vi "Line Intersection With Sprite.vi"(9 "Pixel Data in":u32[][](array[colorbox]), 10 "Line End Point":refnum<class "Vector 2D.lvclass">, 11 "Line Start Point":refnum<class "Vector 2D.lvclass">) -> (2 "Hit Point":refnum<class "Vector 2D.lvclass">, 3 "Hit":bool)   [LabVIEW 2021, in "Collision.lvlib"]
uses:
  Collision.lvlib
  Vector 2D/Vector 2D.lvclass
  Vector 2D/Vector 2D.lvclass/Vector 2D.ctl
panel:
  out "Pixel Data out":u32[][](array[colorbox])
  in  "Colour":u32(colorbox)=16720402
  out "Iteration":i32
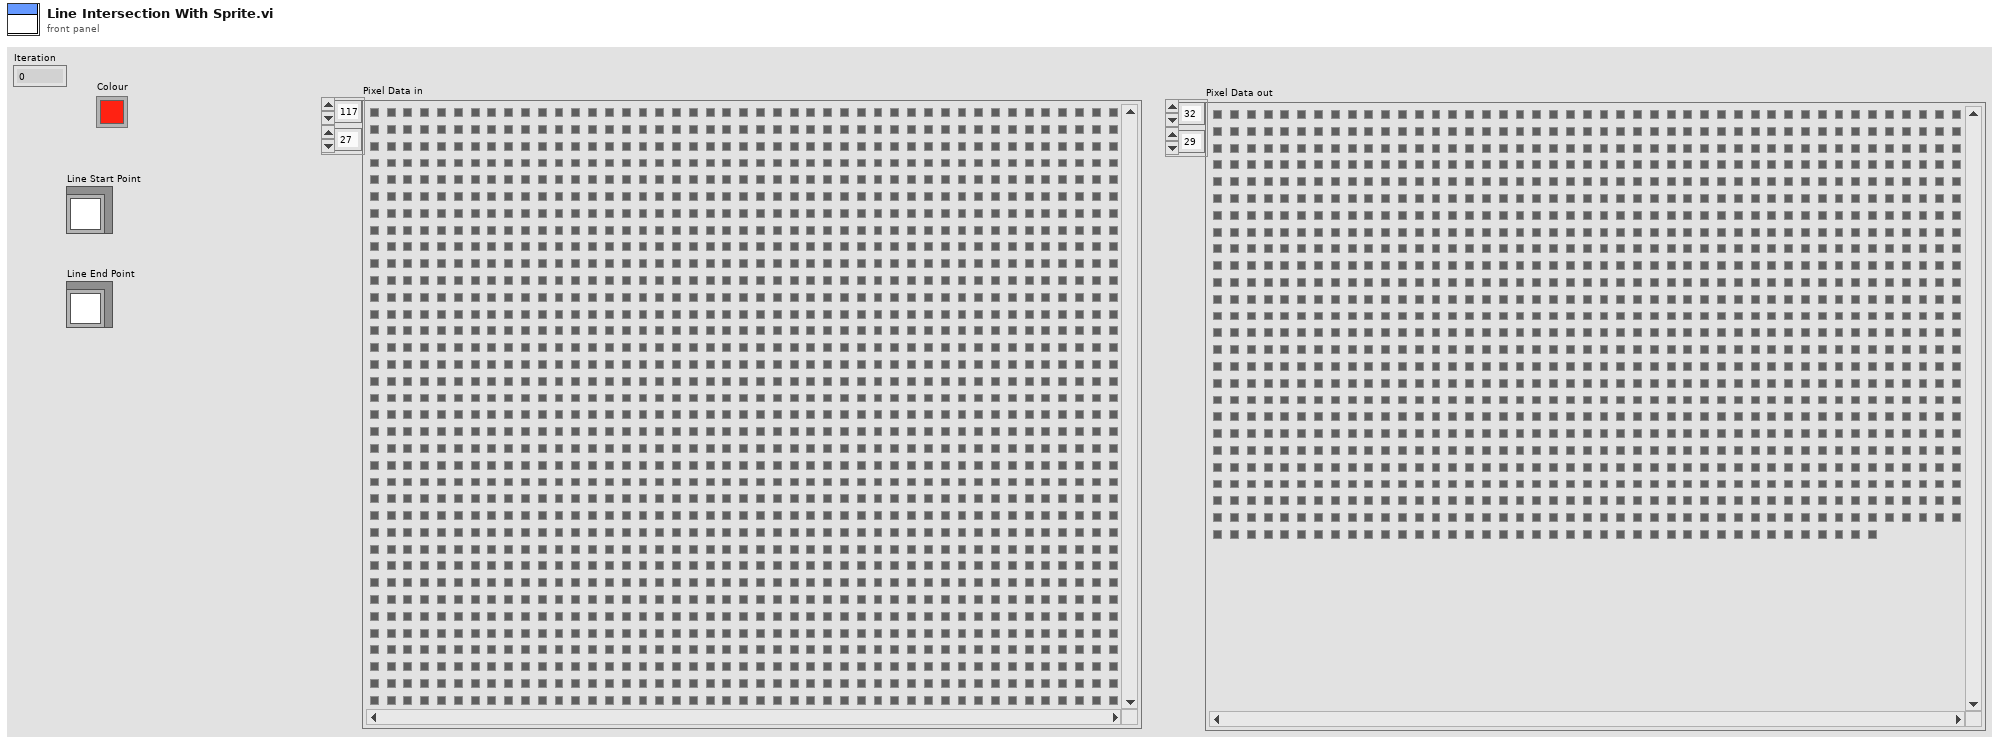
[diagram p1: front panel]
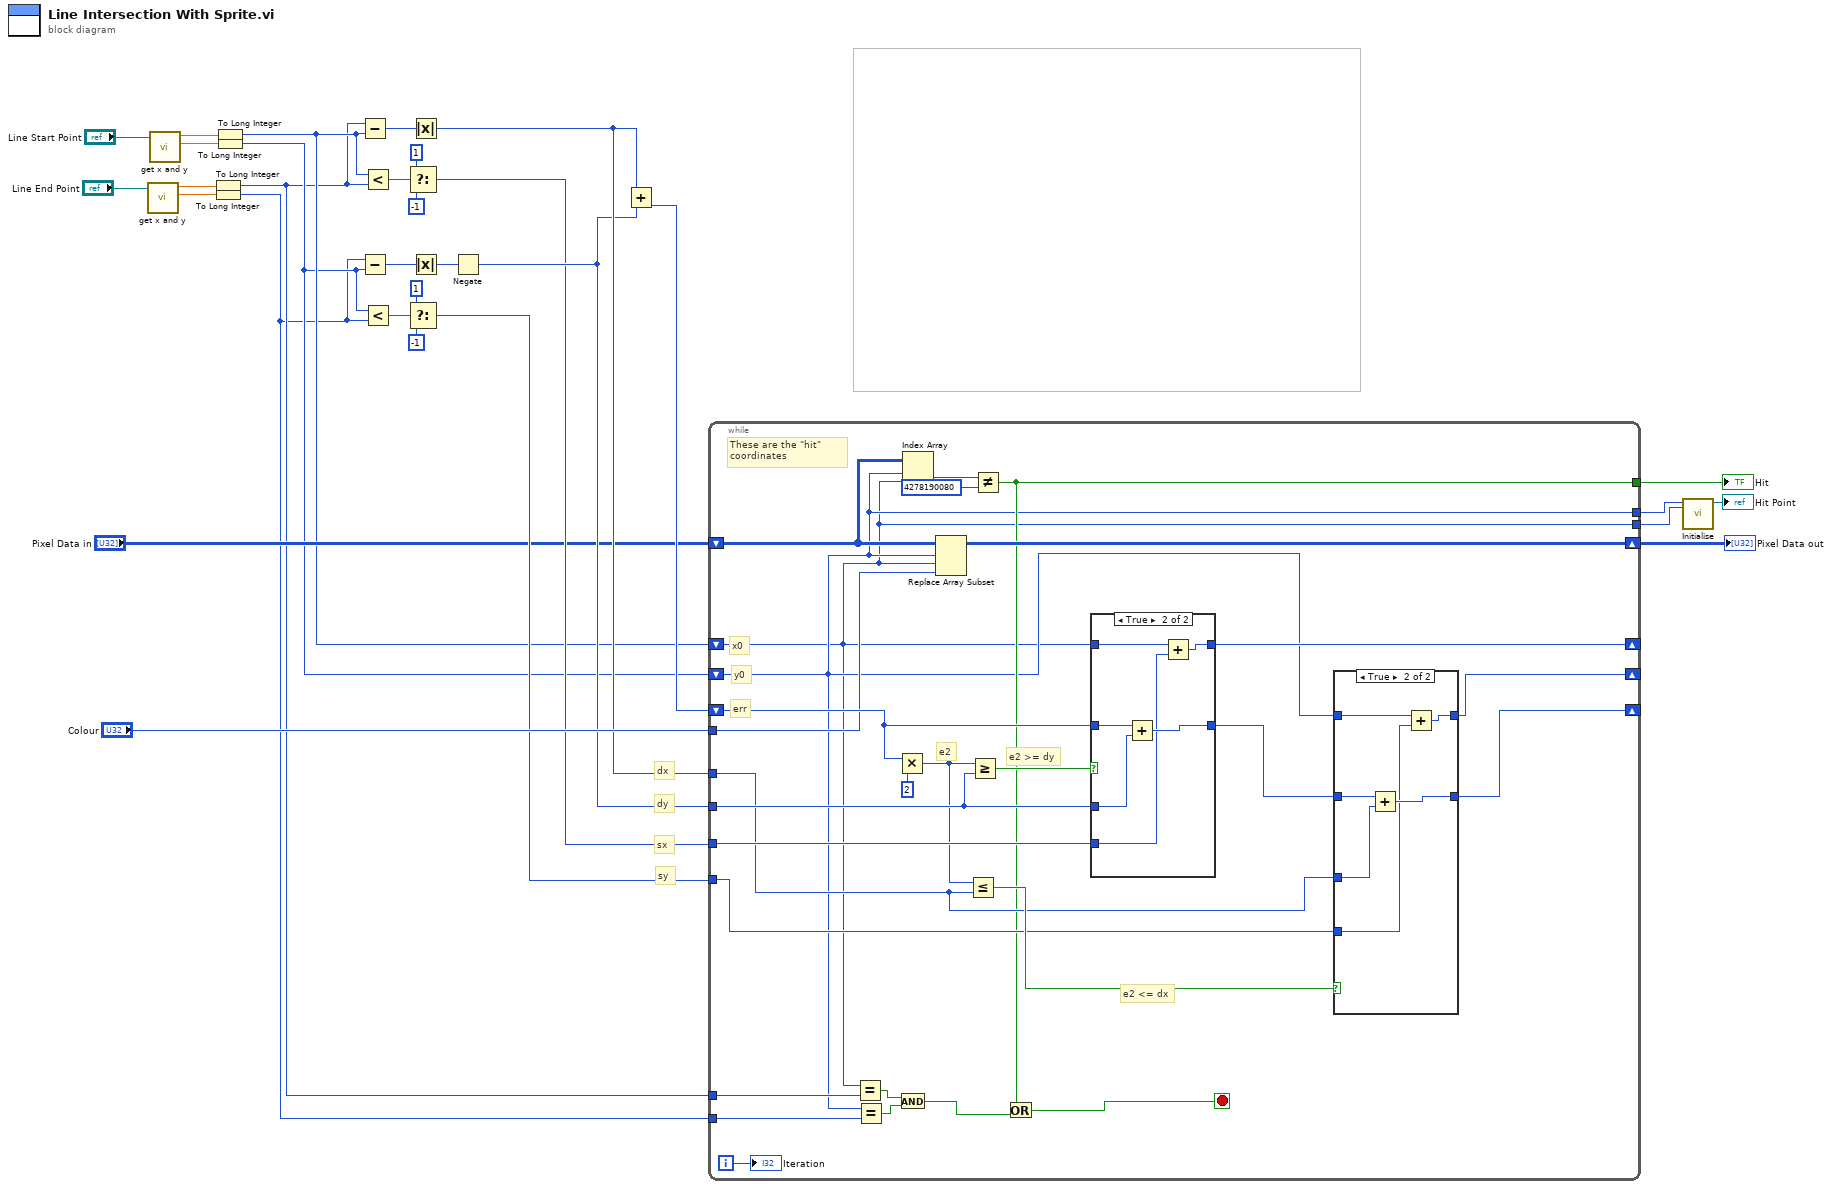
[diagram p0: block diagram]
diagram:
  # "sy"
  # "sx"
  # "dy"
  # "dx"
  n1 = call "get x and y.vi"("Vector 2D in"="Line End Point") -> ("y"=w12:sgl, "x"=w11:sgl)  [unwired: 9 in]
  n2 = call "get x and y.vi"("Vector 2D in"="Line Start Point") -> ("y"=w13:sgl, "x"=w14:sgl)  [unwired: 9 in]
  n3 = To Long Integer(number=w11) -> (32bit integer=w7:i32)
  n4 = To Long Integer(number=w12) -> (32bit integer=w6:i32)
  n5 = To Long Integer(number=w14) -> (32bit integer=w9:i32)
  n6 = To Long Integer(number=w13) -> (32bit integer=w8:i32)
  n7 = Subtract(x=w7, y=w9) -> (x-y=w31:i32)
  n8 = Subtract(x=w6, y=w8) -> (x-y=w24:i32)
  n9 = Less?(x=w9, y=w7) -> (x < y?=w30:bool)
  n10 = Less?(x=w8, y=w6) -> (x < y?=w25:bool)
  n11 = Select(t=1 ("x-y"), s=w30, f=-1 ("x-y")) -> (s? t:f=w18:i32)
  n12 = Select(t=1 ("x-y"), s=w25, f=-1 ("x-y")) -> (s? t:f=w17:i32)
  n13 = Absolute Value(x=w31) -> (abs(x)=w20:i32)
  n14 = Absolute Value(x=w24) -> (abs(x)=w23:i32)
  n15 = Negate(x=w23) -> (-x=w19:i32)
  n16 = Add(x=w20, y=w19) -> (x+y=w21:i32)
  n17 = while {
    shift-right: [w50] -> _
    shift-left: w9 -> [w32]
    shift-right: [w46] -> _
    shift-left: w8 -> [w33]
    tunnel: "Colour" -> [w39]
    tunnel: w7 -> [w59]
    tunnel: w6 -> [w58]
    shift-right: [w44] -> _
    shift-left: w21 -> [w53]
    tunnel: w20 -> [w45]
    tunnel: w19 -> [w52]
    tunnel: w18 -> [w51]
    tunnel: w17 -> [w43]
    shift-right: [w41] -> w5
    shift-left: "Pixel Data in" -> [w40]
    tunnel: [w34] -> w4
    tunnel: [w33] -> w3
    tunnel: [w32] -> w2
    i -> [w42]
    stop <- w35 stop-if-true
    # "These are the \"hit\" coordinates"
    # "e2 <= dx"
    # "e2 >= dy"
    # "e2"
    # "err"
    # "y0"
    # "x0"
    n18 = Equal?(x=w32, y=w59) -> (x = y?=w57:bool)
    n19 = Equal?(x=w33, y=w58) -> (x = y?=w56:bool)
    n20 = Multiply(x=w53, y=2) -> (x*y=w49:i32)
    n21 = And(x=w57, y=w56) -> (x .and. y?=w36:bool)
    n22 = Index Array(array=w40, index (row)=w33, index (col)=w32) -> (element=w38:u32)
    n23 = Replace Array Subset(array=w40, new element=w39, index (row)=w33, index (col)=w32) -> (w41:u32[][])
    n24 = Less Or Equal?(x=w49, y=w45) -> (x <= y?=w48:bool)
    n25 = Greater Or Equal?(x=w49, y=w52) -> (x >= y?=w54:bool)
    n26 = Not Equal?(x=w38, y=u32 4278190080) -> (x != y?=w34:bool)
    n27 = Or(x=w34, y=w36) -> (x .or. y?=w35:bool)
    n28 = case shown="True" w54 {
      tunnel: w53 -> [w60 w67]
      tunnel: w52 -> [_ w66]
      tunnel: [w60 w65] -> w47
      tunnel: w32 -> [w61 w64]
      tunnel: w51 -> [_ w63]
      tunnel: [w61 w62] -> w50
      frame False {
      }
      frame True {
        n29 = Add(x=w67, y=w66) -> (x+y=w65:i32)
        n30 = Add(x=w64, y=w63) -> (x+y=w62:i32)
      }
    }
    n31 = case shown="True" w48 {
      tunnel: w47 -> [w69 w75]
      tunnel: w45 -> [_ w74]
      tunnel: [w69 w73] -> w44
      tunnel: w33 -> [w68 w72]
      tunnel: w43 -> [_ w71]
      tunnel: [w68 w70] -> w46
      frame False {
      }
      frame True {
        n32 = Add(x=w75, y=w74) -> (x+y=w73:i32)
        n33 = Add(x=w72, y=w71) -> (x+y=w70:i32)
      }
    }
    "Iteration" <- w42
  }
  "Pixel Data out" <- w5
  "Hit" <- w4
  n34 = call "Initialise.vi"("y"=w2, "x"=w3) -> ("Vector 2D out"=→"Hit Point":refnum<class "Vector 2D.lvclass">)  [unwired: 9 in]
